vi "Main.vi"() -> ()   [LabVIEW 2017]
doc: "The myRIO Project template acquires acceleration data from the onboard accelerometer and displays the changes of acceleration values in a waveform chart."
uses:
  <vilib>/Platform/TimedLoop/XDataNode/timing_clust.ctl
  <vilib>/Platform/TimedLoop/XDataNode/nitl_modes.ctl
  <vilib>/Platform/TimedLoop/XDataNode/wakeup.ctl
  <vilib>/FPGAPlugInAG/myRIO-1900/niLvFpga_Open_myRIO-1900.vi
  <vilib>/rvi/interface/common/dynamic/niFpgaDynamicAddResources.vi
  <vilib>/myRIO/Common/Instrument Driver Framework/Utilities/vis/FPGA Ref Manager.vi
  <vilib>/Utility/error.llb/Error Cluster From Error Code.vi
  <vilib>/myRIO/Common/Instrument Driver Framework/Utilities/vis/Ref Counter.vi
  <vilib>/rvi/errors/niLvFpgaAdjustHostInterfaceError.vi
  <vilib>/imath/engines/lvmath2/RunTimeEngine/NodeEndStatement/NIMS_NodeEndStatement_Output.vi
  <instcachedir>/0/NIMS_NodeEndStatement_Output_53EC0D466D134D7ABD903AC30B43404B.lvgen/NIMS_NodeEndStatement_Output_53EC0D466D134D7ABD903AC30B43404B_001.vi
  <vilib>/imath/engines/lvmath2/RunTimeEngine/ErrorHandling/NIMS_Finalize Error.vi
  <vilib>/FPGAPlugInAG/Dynamic/niLvFpga_Close_Dynamic.vi
  <vilib>/rvi/interface/nirviOpenFPGA/nirviOpenFPGA.xnode
  FPGA Bitfiles/FPGADEMO_FPGATarget_FPGAENCODER_hVHewW9304I.lvbitx
  <vilib>/platform/TimedLoop/XDataNode/XDataNode.xnode
  <vilib>/rvi/interface/nirviReadWriteControl/nirviReadWriteControl.xnode
  <vilib>/rvi/interface/nirviCloseFPGA/nirviCloseFPGA.xnode
  <vilib>/Platform/TimedLoop/XDataNode/XDNodeRunTimeDep.lvlib
  <vilib>/myRIO/Instrument Drivers/Utilities/Utilities.lvlib
  NiFpgaLv.dll
  <vilib>/rvi/interface/Simulation/niFpgaSimulationCallBeginRW.vi
panel:
  in  "coeff_Hz":dbl
  out "r/min_Hz":i32
  in  "coeff_T":dbl
  out "r/min_T":u32
  out "Waveform Chart 2":cluster{dbl, dbl, dbl}[](graph)
  in  "Filter Counts":u16
  in  "Clear Overflow?":bool
  in  "Clear Error?":bool
  in  "Reset":bool
  in  "Pause?":bool
  in  "Clear Sigam?":bool
  in  "Reference Input":T1={"Amp"=0.0, "Fred"=0.01, "Offset"=0.0, "Type"=0.0} {"Offset" step=0.1; "Fred" min=0.001 step=0.1; "Amp" step=0.1}
  in  "PID Parameters":cluster{"Kp":dbl, "Ki":dbl, "Kd":dbl} {"Kd" step=0.1; "Ki" step=0.1; "Kp" step=0.1}
  in  "stop":bool
  out "error out":errorcluster
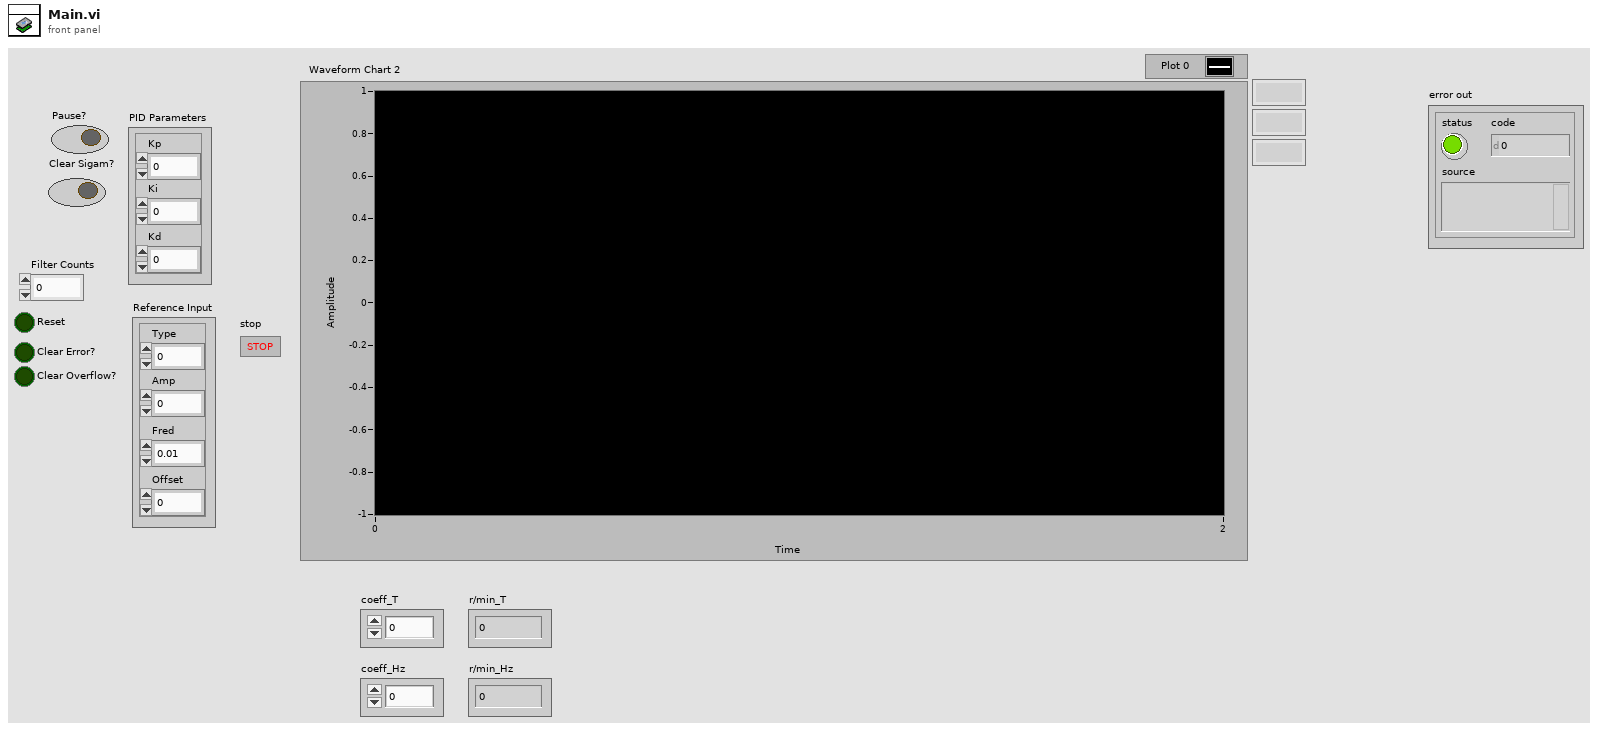
[diagram p1: front panel]
types:
  T1 = cluster{"Amp":dbl, "Fred":dbl, "Offset":dbl, "Type":dbl}
  T2 = typedef "XDNodeRunTimeDep.lvlib/timing_clust.ctl" = cluster{"Expected End [f-1]":u64, "Actual End [f-1]":u64, "Finished Late? [f-1]":bool, "Expected End [i-1]":u64, "Actual End [i-1]":u64, "Finished Late? [i-1]":bool, "Expected Start [i]":u64, "Actual Start [i]":u64, "Expected Start [f]":u64, "Actual Start [f]":u64, "Source Name":string, "Structure Name":string, "Period":i64, "Deadline":i64, "Offset":i64, "Start":i64, "Priority":i32, "Timeout":i32, "Mode":T3, "Wakeup Reason":T4, "Error":errorcluster, "Source Type":string, "Secondary Source Type":string, "Global End Time":u64, "Global Start Time":u64, "Frame Duration":u64, "Iteration Duration":u64, "Assigned CPU":i32, "I/O Scan Engine Mode":u32}
  T3 = typedef "XDNodeRunTimeDep.lvlib/nitl_modes.ctl" = enum32{"No Change", "Process missed periods, maintain original phase", "Discard missed periods, maintain original phase", "Process missed periods, ignore original phase", "Discard missed periods, ignore original phase"}
  T4 = typedef "XDNodeRunTimeDep.lvlib/wakeup.ctl" = enum32{"Normal", "Aborted", "Asynchronous wakeup", "Timing source error", "Timed loop error", "Timeout"}
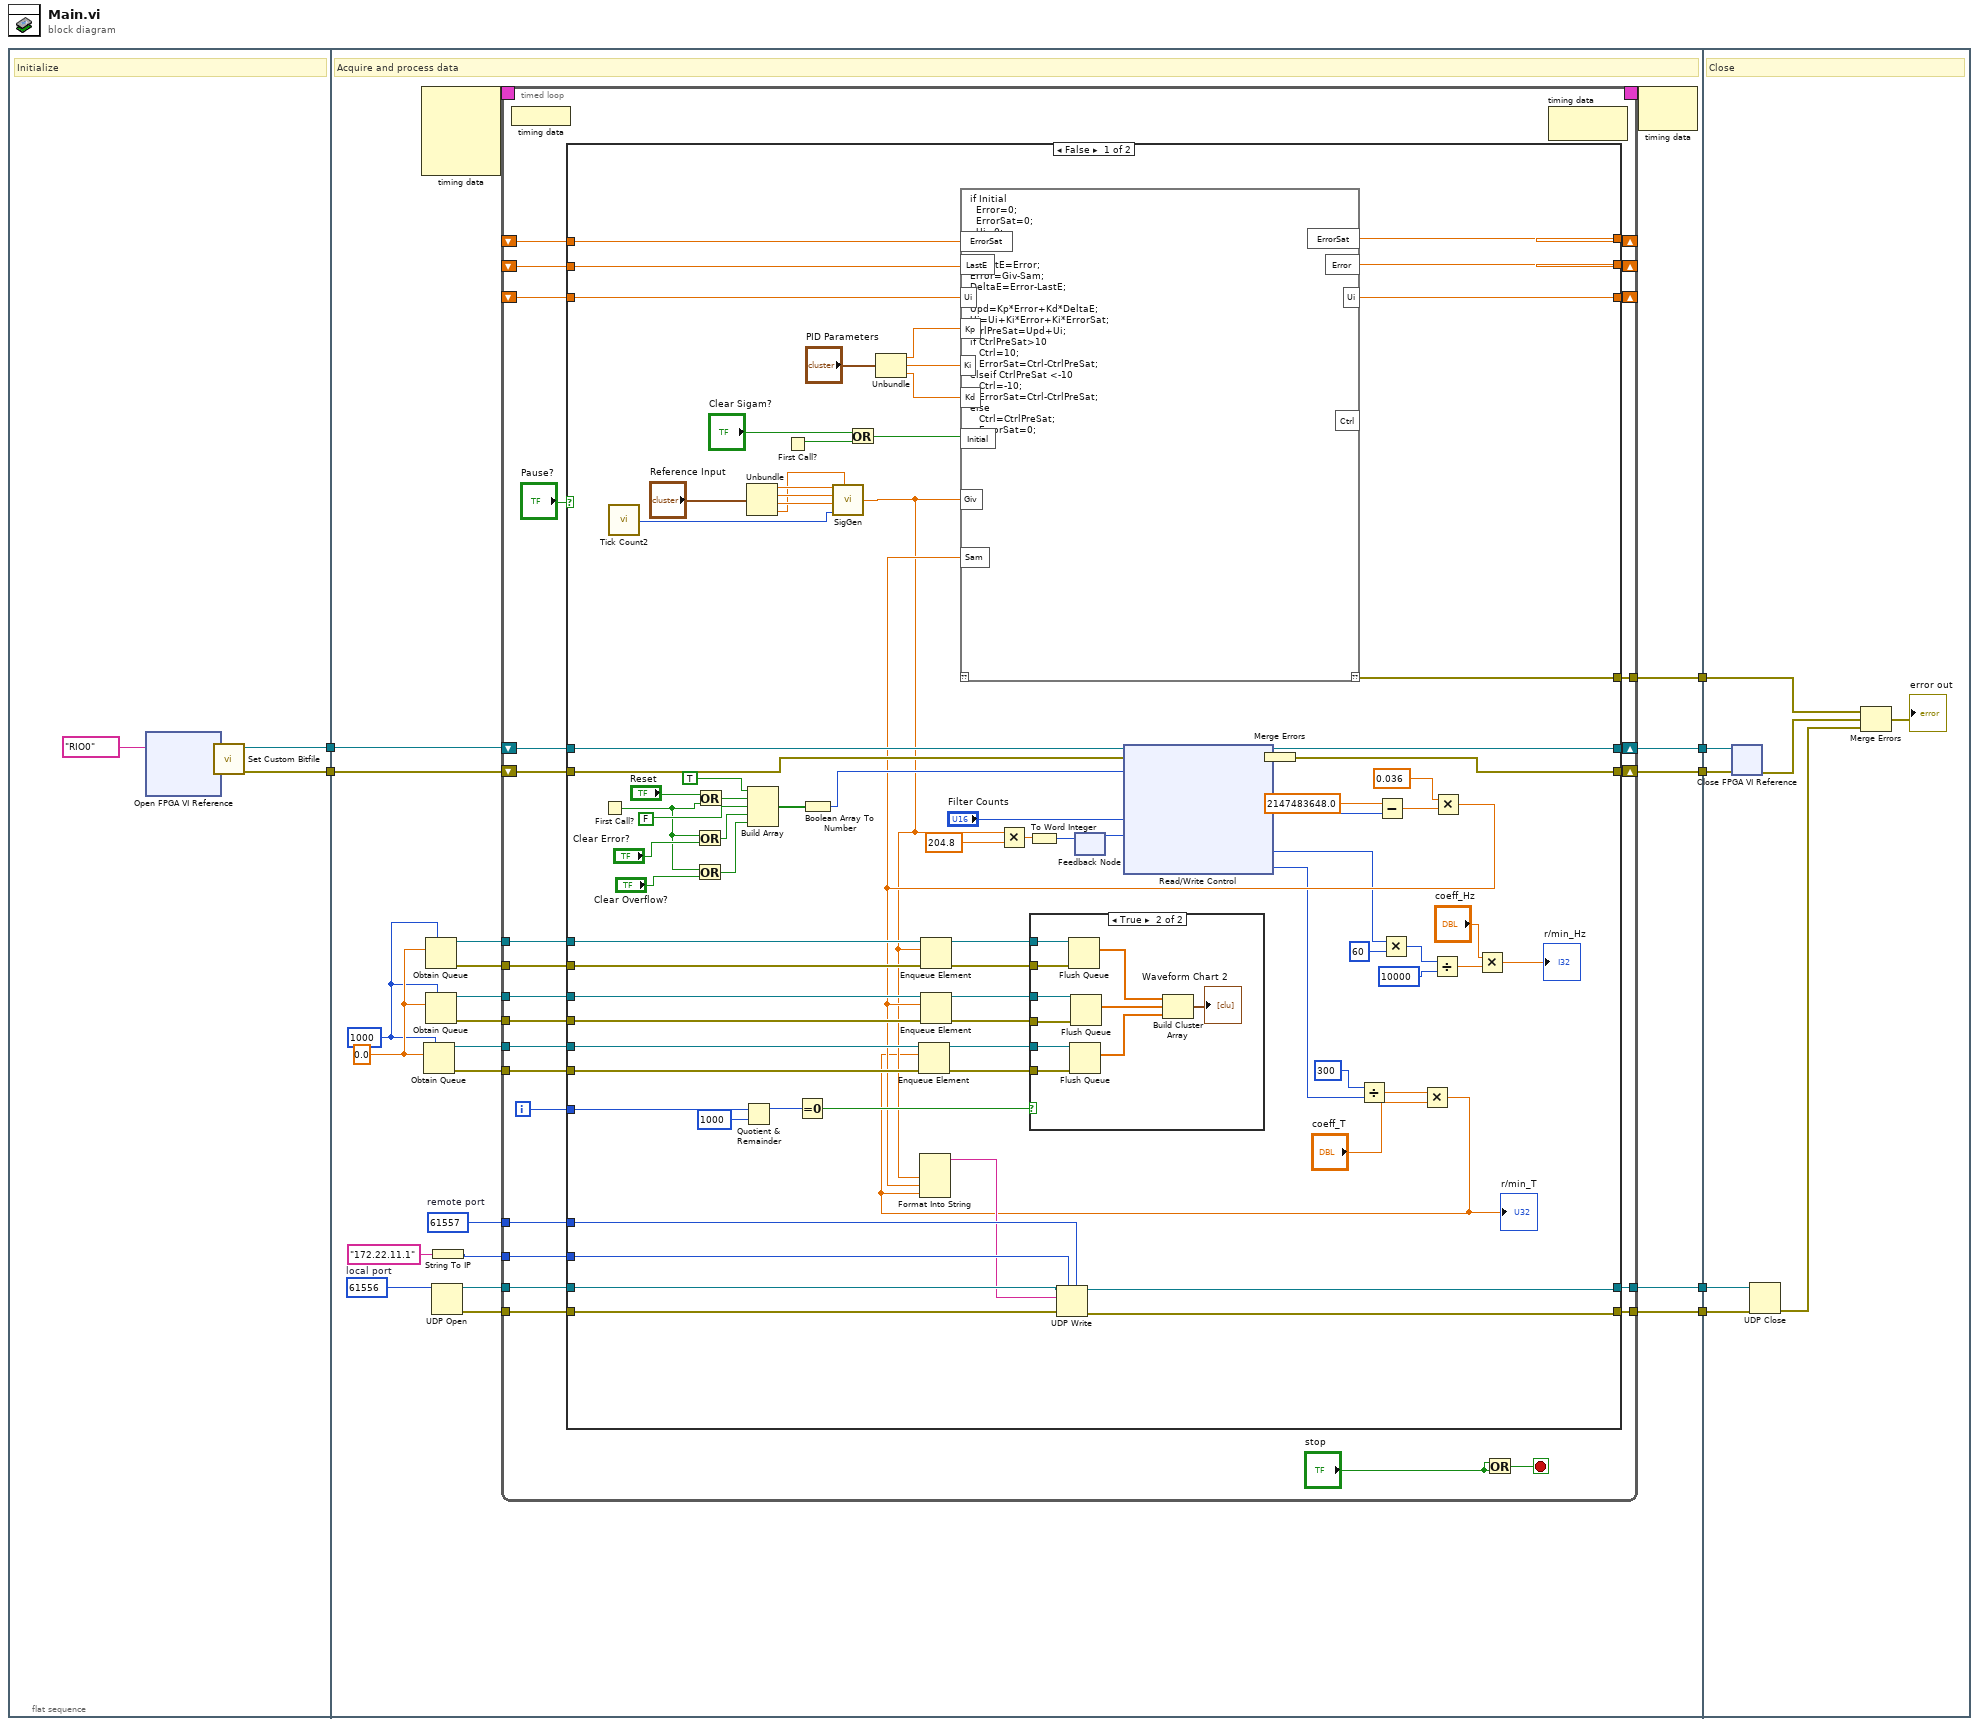
[diagram p0: block diagram]
diagram:
  n1 = flat-sequence {
    tunnel: [w9] -> w7
    tunnel: [w8] -> w6
    tunnel: w7 -> [w33]
    tunnel: w6 -> [w32]
    tunnel: [w31] -> w5
    tunnel: [w30] -> w4
    tunnel: [w29] -> w3
    tunnel: [w14] -> w2
    tunnel: [w13] -> w1
    tunnel: w5 -> [w344]
    tunnel: w4 -> [w343]
    tunnel: w3 -> [w341]
    tunnel: w2 -> [w340]
    tunnel: w1 -> [w339]
    frame #0 {
      # "Initialize"
      n2 = xnode "Open FPGA VI Reference"("resource name"=tag "RIO0") -> ("FPGA VI Reference Out"=w10:refnum<k20>, "error out"=w11:errorcluster)  [unwired: 1 in]
      n3 = call <vilib>:"Set Custom Bitfile.vi"("error in (no error)"=w11, "Custom FPGA Reference In"=w10) -> ("error out"=w8:errorcluster, "Custom FPGA Reference Out"=w9:refnum<k20>)  [unwired: 8 in]
    }
    frame #1 {
      w15 = u16 61557  # remote port
      w20 = u16 61556  # local port
      w26 = 0.0
      w25 = 1000 ("max queue size (-1, unlimited)")
      # "Acquire and process data"
      n4 = node-c288() -> (w35:T2)  [unwired: 4 in]
      n5 = Obtain Queue(max queue size (-1, unlimited)=w25, element data type=w26) -> (queue out=w28:refnum<queue>, error out=w27:errorcluster)  [unwired: 3 in, 1 out]
      n6 = Obtain Queue(max queue size (-1, unlimited)=w25, element data type=w26) -> (queue out=w23:refnum<queue>, error out=w22:errorcluster)  [unwired: 3 in, 1 out]
      n7 = Obtain Queue(max queue size (-1, unlimited)=w25, element data type=w26) -> (queue out=w24:refnum<queue>, error out=w21:errorcluster)  [unwired: 3 in, 1 out]
      n8 = UDP Open(11:w20) -> (port=w17:refnum<k16>, 0:w16:errorcluster)  [unwired: 4 in, 1 out]
      n9 = String To IP(1:"172.22.11.1" ("name")) -> (0:w19:u32)
      n10 = timed-loop {
        timing: w35 -> [_]
        timing-out: [_] -> w34
        shift-right: [w57] -> _
        shift-left: _ -> [w62]
        shift-right: [w61] -> _
        shift-left: _ -> [w60]
        shift-right: [w59] -> _
        shift-left: _ -> [w58]
        shift-right: [w50] -> w31
        shift-left: w33 -> [w53]
        shift-right: [w51] -> w30
        shift-left: w32 -> [w52]
        tunnel: [w49] -> w29
        tunnel: w28 -> [w47]
        tunnel: w27 -> [w46]
        tunnel: w24 -> [w45]
        tunnel: w23 -> [w44]
        tunnel: w22 -> [w43]
        tunnel: w21 -> [w42]
        tunnel: w19 -> [w41]
        tunnel: w17 -> [w40]
        tunnel: w16 -> [w39]
        tunnel: w15 -> [w38]
        tunnel: [w37] -> w14
        tunnel: [w36] -> w13
        i -> [w48]
        stop <- w56 stop-if-true
        n11 = node-c288() -> ()  [unwired: 1 in]
        n12 = case shown="False" "Pause?" {
          tunnel: w62 -> [w140 w331]
          tunnel: [w139 w332] -> w61
          tunnel: w60 -> [w138 w332]
          tunnel: [w137 w333] -> w59
          tunnel: w58 -> [w136 w333]
          tunnel: [w132 w331] -> w57
          tunnel: w53 -> [w130 w330]
          tunnel: w52 -> [w129 w329]
          tunnel: [w112 w329] -> w51
          tunnel: [w111 w330] -> w50
          tunnel: [w110 _] -> w49
          tunnel: w48 -> [w109 _]
          tunnel: w47 -> [w95 _]
          tunnel: w46 -> [w94 _]
          tunnel: w45 -> [w91 _]
          tunnel: w44 -> [w90 _]
          tunnel: w43 -> [w89 _]
          tunnel: w42 -> [w88 _]
          tunnel: w41 -> [w80 _]
          tunnel: w40 -> [w82 w328]
          tunnel: w39 -> [w81 w327]
          tunnel: w38 -> [w79 _]
          tunnel: [w77 w328] -> w37
          tunnel: [w76 w327] -> w36
          frame False {
            n13 = First Call?() -> (First Call?: T/F=w122:bool)
            n14 = call "Tick Count2"() -> ("Tick Count(uSec)"=w131:u32)
            n15 = Or(x=w122, y="Clear Error?") -> (x .or. y?=w121:bool)
            n16 = Or(x=w122, y="Clear Overflow?") -> (x .or. y?=w120:bool)
            n17 = Or(x="Reset", y=w122) -> (x .or. y?=w127:bool)
            n18 = Quotient & Remainder(x=w109, y=1000) -> (x-y*floor(x/y)=w106:i32)  [unwired: 1 out]
            n19 = Unbundle("Reference Input") -> ("Amp"=w99:dbl, "Fred"=w98:dbl, "Offset"=w97:dbl, "Type"=w96:dbl)
            n20 = Build Array(TRUE, w127, FALSE, w121, w120) -> (w119:bool[])
            n21 = First Call?() -> (First Call?: T/F=w133:bool)
            n22 = Equal To 0?(x=w106) -> (x = 0?=w107:bool)
            n23 = Boolean Array To Number(Boolean array=w119) -> (number=w118:u32)
            n24 = call "SigGen.vi"("Amp"=w99, "Freq"=w98, "Offset"=w97, "Timer"=w131, "Type"=w96) -> ("Output"=w64:dbl)
            n25 = Or(x="Clear Sigam?", y=w133) -> (x .or. y?=w135:bool)
            n26 = Unbundle("PID Parameters") -> ("Kp"=w143:dbl, "Ki"=w142:dbl, "Kd"=w141:dbl)
            n27 = Enqueue Element(queue=w90, element=w64, error in (no error)=w89) -> (queue out=w85:refnum<queue>, error out=w86:errorcluster)  [unwired: 1 in, 1 out]
            n28 = Multiply(x=w64, y=204.8) -> (x*y=w105:dbl)
            n29 = To Word Integer(number=w105) -> (16bit integer=w102:i16)
            n30 = feedback-in #1(w102) -> ()
            n31 = feedback #1() -> (w101:i16)  [unwired: 1 in]
            n32 = xnode "Read/Write Control"("FPGA VI Reference In"=w130, "error in"=w129, "CNFG"=w118, "Debounce Ticks"="Filter Counts", "ConnectorC/AO1"=w101) -> ("FPGA VI Reference Out"=w111:refnum<k20>, "error out"=w117:errorcluster, "CNTR"=w113:u32, "Pulses/Millisecond"=w71:i32, "*2.5E-8 Second/Period"=w75:u32)  [unwired: 1 out]
            n33 = Merge Errors(w117) -> (w112:errorcluster)
            n34 = Divide(x=u32 300, y=w75) -> (x/y=w73:dbl)
            n35 = Subtract(x=2147483648.0, y=w113) -> (x-y=w115:dbl)
            n36 = Multiply(x=w71, y=60) -> (x*y=w69:i32)
            n37 = Multiply(x=w73, y="coeff_T") -> (x*y=w63:dbl)
            "r/min_T" <- w63
            n38 = Enqueue Element(queue=w95, element=w63, error in (no error)=w94) -> (queue out=w93:refnum<queue>, error out=w92:errorcluster)  [unwired: 1 in, 1 out]
            n39 = Divide(x=w69, y=10000) -> (x/y=w67:dbl)
            n40 = Multiply(x=0.036, y=w115) -> (x*y=w83:dbl)
            n41 = Format Into String(w64, w83, w63) -> (resulting string=w78:string)  [unwired: 3 in, 1 out]
            n42 = Enqueue Element(queue=w91, element=w83, error in (no error)=w88) -> (queue out=w84:refnum<queue>, error out=w87:errorcluster)  [unwired: 1 in, 1 out]
            n43 = mathscript code="if Initial\n  Error=0;\n  ErrorSat=0;\n  Ui=0;\nend;\n\n%LastE=Error;\nError=Giv-Sam;\nDeltaE=Error-LastE;\n\nUpd=Kp*Error+Kd*DeltaE;\nUi=Ui+Ki*Error+Ki*ErrorSat;\nCtrlPreSat=Upd+Ui;\nif CtrlPreSat>10\n   Ctrl=10;\n   ErrorSat=Ctrl-CtrlPreSat;\nelseif CtrlPreSat <-10\n   Ctrl=-10;\n   ErrorSat=Ctrl-CtrlPreSat;\nelse \n   Ctrl=CtrlPreSat;\n   ErrorSat=0;\nend;"("Giv"=w64, "Sam"=w83, "Kp"=w143, "Ki"=w142, "Kd"=w141, "Ui"=w140, "Initial"=w135, "LastE"=w138, "ErrorSat"=w136) -> ("??"=w110:errorcluster, "Ui"=w132:dbl, "Error"=w139:dbl, "ErrorSat"=w137:dbl)  [unwired: 1 in, 1 out]
            n44 = case shown="True" w107 {
              tunnel: w93 -> [_ w154]
              tunnel: w92 -> [_ w153]
              tunnel: w87 -> [_ w152]
              tunnel: w86 -> [_ w151]
              tunnel: w85 -> [_ w150]
              tunnel: w84 -> [_ w149]
              frame False {
              }
              frame True {
                n45 = Flush Queue(queue=w150, error in (no error)=w151) -> (remaining elements=w147:dbl[])  [unwired: 2 out]
                n46 = Flush Queue(queue=w154, error in (no error)=w153) -> (remaining elements=w145:dbl[])  [unwired: 2 out]
                n47 = Flush Queue(queue=w149, error in (no error)=w152) -> (remaining elements=w148:dbl[])  [unwired: 2 out]
                n48 = Build Cluster Array(w147, w148, w145) -> (→"Waveform Chart 2":cluster{dbl, dbl, dbl}[])
              }
            }
            n49 = UDP Write(address=w80, port or service name=w79, connection ID=w82, data in=w78, 8:w81) -> (error out=w76:errorcluster, 3:w77:refnum<k16>)  [unwired: 1 in]
            n50 = Multiply(x="coeff_Hz", y=w67) -> (x*y=→"r/min_Hz":dbl)
          }
          frame True {
          }
        }
        n51 = Or(x="stop", y="stop") -> (x .or. y?=w56:bool)
        n52 = node-c288() -> ()  [unwired: 1 in, 1 out]
      }
      n53 = node-c288(w34) -> ()  [unwired: 1 out]
    }
    frame #2 {
      # "Close"
      n54 = xnode "Close FPGA VI Reference"("FPGA VI Reference In"=w344, "error in"=w343) -> ("error out"=w342:errorcluster)
      n55 = UDP Close(connection ID=w340, 8:w339) -> (error out=w338:errorcluster)  [unwired: 1 out]
      n56 = Merge Errors(w341, w342, w338) -> (→"error out":errorcluster)
    }
  }
